vi "GDSIconEditor_SplitNameInRows.vi"(1 "name":string) -> (0 "result string":string)   [LabVIEW 2012]
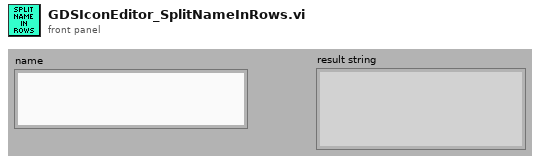
[diagram p1: front panel]
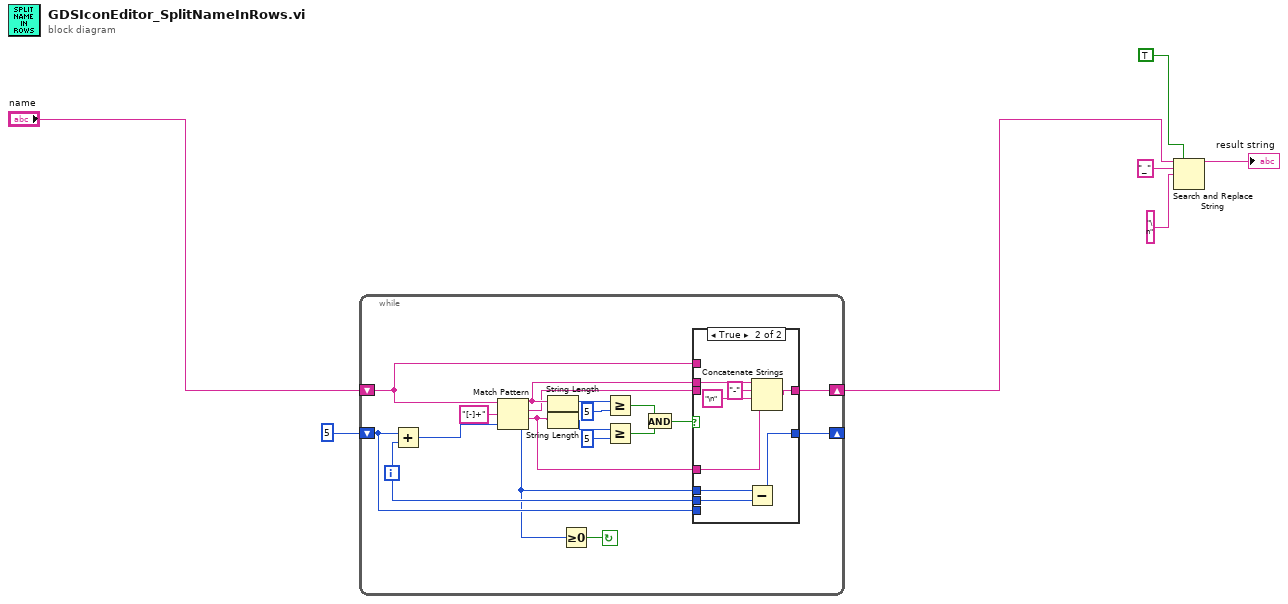
[diagram p0: block diagram]
diagram:
  n1 = while {
    shift-right: [w18] -> w1
    shift-left: "name" -> [w17]
    shift-right: [w11] -> _
    shift-left: 5 -> [w10]
    i -> [w12]
    stop <- w8 continue-if-true
    n2 = Add(x=w10, y=w12) -> (x+y=w16:i32)
    n3 = Match Pattern(string=w17, regular expression="[-]+", offset (0)=w16) -> (before substring=w15:string, match substring=w14:string, after substring=w13:string, offset past match=w9:i32)
    n4 = String Length(string=w15) -> (length=w25:i32)
    n5 = String Length(string=w13) -> (length=w23:i32)
    n6 = Greater Or Equal To 0?(x=w9) -> (x >= 0?=w8:bool)
    n7 = Greater Or Equal?(x=w25, y=5) -> (x >= y?=w21:bool)
    n8 = Greater Or Equal?(x=w23, y=5) -> (x >= y?=w20:bool)
    n9 = And(x=w21, y=w20) -> (x .and. y?=w19:bool)
    n10 = case shown="True" w19 {
      tunnel: w17 -> [w28 _]
      tunnel: [w28 w33] -> w18
      tunnel: w15 -> [_ w36]
      tunnel: w14 -> [_ _]
      tunnel: w13 -> [_ w34]
      tunnel: w9 -> [_ w32]
      tunnel: w12 -> [_ w31]
      tunnel: [w27 w30] -> w11
      tunnel: w10 -> [w27 _]
      frame False {
      }
      frame True {
        n11 = Subtract(x=w32, y=w31) -> (x-y=w30:i32)
        n12 = Concatenate Strings(w36, "-" ("string"), "\n" ("string"), w34) -> (w33:string)
      }
    }
  }
  n13 = Search and Replace String(replace all?=TRUE ("replace all? (F)"), input string=w1, search string="_", replace string="\n" ("replace string (\"\")")) -> (result string=→"result string":string)  [unwired: 4 in, 3 out]
